vi "getSyncedTone.vi"(8 "error in":errorcluster, 10 "signal":waveform(dbl), 11 "sync-state":enum16{"not-sync", "synced"}(ring)) -> (0 "error out":errorcluster, 1 "tone":i32, 2 "sync?":bool, 3 "sync-state":enum16{"not-sync", "synced"}(ring))   [LabVIEW 2013]
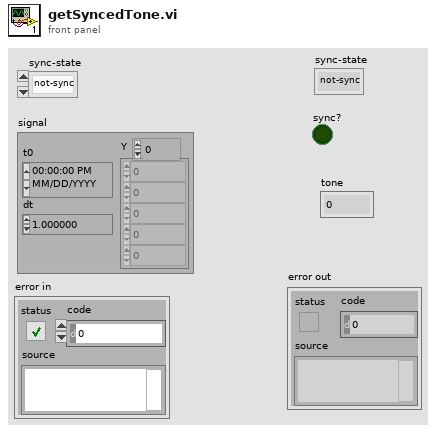
[diagram p1: front panel]
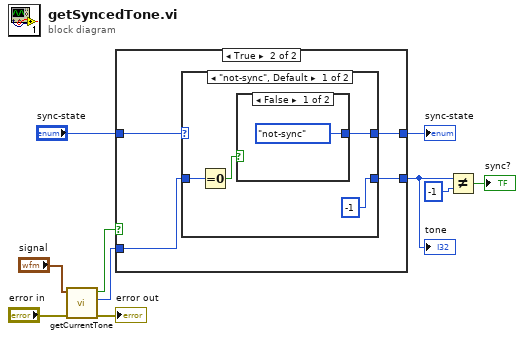
[diagram p0: block diagram]
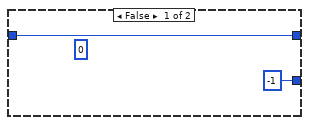
[diagram p2: hidden frame]
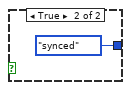
[diagram p3: hidden frame]
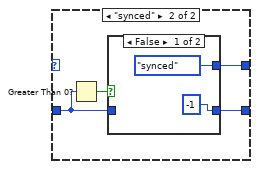
[diagram p4: hidden frame]
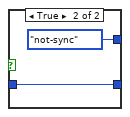
[diagram p5: hidden frame]
diagram:
  n1 = call "getCurrentTone.vi"("error in"="error in", "signal"="signal") -> ("error out"=→"error out":errorcluster, "tone"=w7:i32, "vaild?"=w6:bool)  [unwired: 7 in]
  n2 = case shown="True" w6 {
    tunnel: w7 -> [_ w14]
    tunnel: [-1 w13] -> w5
    tunnel: "sync-state" -> [w12 w16]
    tunnel: [w12 w15] -> w10
    frame False {
      (unwired) 0
    }
    frame True {
      n3 = case shown="\"not-sync\", Default" w16 {
        tunnel: w14 -> [w20 w24]
        tunnel: [w18 w25] -> w15
        tunnel: [-1 w23] -> w13
        frame "not-sync", Default {
          n4 = Equal To 0?(x=w20) -> (x = 0?=w19:bool)
          n5 = case shown="False" w19 {
            tunnel: [enum16{"not-sync", "synced"}."not-sync" enum16{"not-sync", "synced"}."synced"] -> w18
            frame False {
            }
            frame True {
            }
          }
        }
        frame "synced" {
          n6 = Greater Than 0?(x=w24) -> (x > 0?=w26:bool)
          n7 = case shown="False" w26 {
            tunnel: [enum16{"not-sync", "synced"}."synced" enum16{"not-sync", "synced"}."not-sync"] -> w25
            tunnel: w24 -> [_ w29]
            tunnel: [-1 w29] -> w23
            frame False {
            }
            frame True {
            }
          }
        }
      }
    }
  }
  "sync-state" <- w10
  "tone" <- w5
  n8 = Not Equal?(x=w5, y=-1) -> (x != y?=→"sync?":bool)
